vi "OA Get Mode Acq Params.vi"(10 "pcListOfParams":string, 11 "pcModeName":string) -> (2 "pcListOfParams out":string, 3 "function return":u32)   [LabVIEW 2018, in "Copy of Andor SDK.lvlib"]
doc: "EXPNETTYPE unsigned int WINAPI OA_GetModeAcqParams(const char * const pcModeName, char * const pcListOfParams);"
uses:
  Copy of Andor SDK.lvlib
  <userlib>/Andor SDK/ATMCD32D.dll
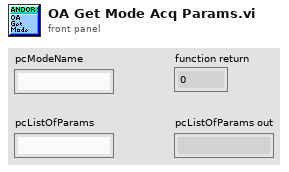
[diagram p1: front panel]
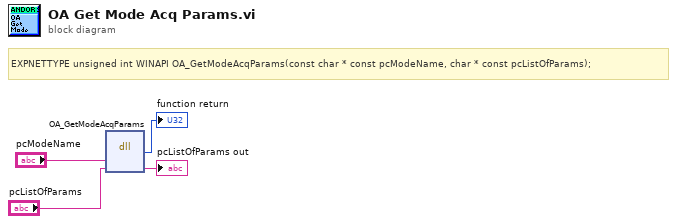
[diagram p0: block diagram]
diagram:
  # "EXPNETTYPE unsigned int WINAPI OA_GetModeAcqParams(const char * const pcModeName, char * const pcListOfParams);"
  n1 = dll-call lib="C:/Program Files (x86)/National Instruments/LabVIEW 2018/user.lib/Andor SDK/ATMCD32D.*" fn="OA_GetModeAcqParams"("pcModeName"="pcModeName", "pcListOfParams"="pcListOfParams") -> (→"function return":u32, "pcListOfParams"=→"pcListOfParams out":string)  [unwired: 4 in, 2 out]
